vi "Format Numeric to String.vi"(6 "Numeric":dbl, 7 "Endian":T1, 8 "Format String":string, 9 "List":string[](array[string]), 10 "Channel Type":T2, 11 "Type":T3) -> (3 "Value":string)   [LabVIEW 2018, in "Instrument Addon Engine.lvlib"]
uses:
  Instrument Addon Engine.lvlib
  Addon Shared/Types/Type Cast Type.ctl
  Addon Shared/Types/Metadata Channel Type.ctl
  Addon Shared/Types/Endian.ctl
  Addon Shared/Instrument Addon Shared.lvlib
panel:
  in  "error in":errorcluster
  out "error out":errorcluster
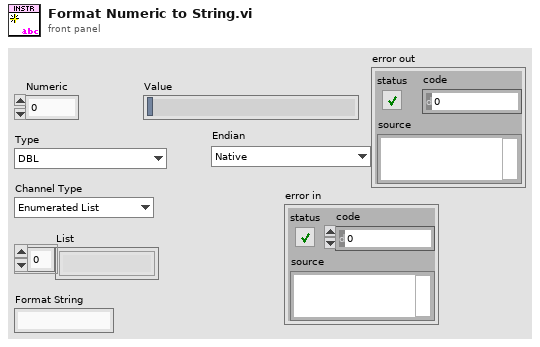
[diagram p1: front panel]
types:
  T1 = typedef "Instrument Addon Shared.lvlib/Endian.ctl" = enum16{"Native", "Little", "Big"}
  T2 = typedef "Instrument Addon Shared.lvlib/Metadata Channel Type.ctl" = enum16{"Enumerated List", "Format", "Type Cast"}
  T3 = typedef "Instrument Addon Shared.lvlib/Type Cast Type.ctl" = enum16{"DBL", "SGL", "U64", "U32", "U16", "U8", "I64", "I32", "I16", "I8"}
  T4 = enum16{"big-endian, network order", "native, host order", "little-endian"}
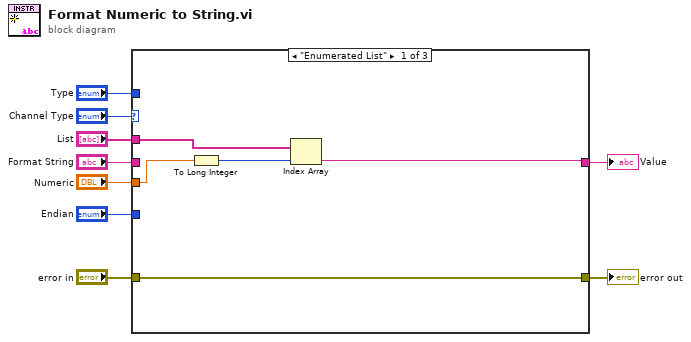
[diagram p0: block diagram]
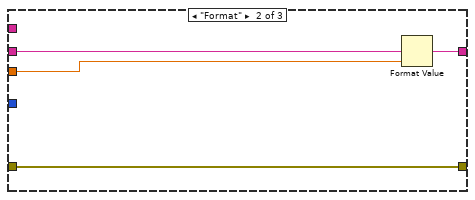
[diagram p2: hidden frame]
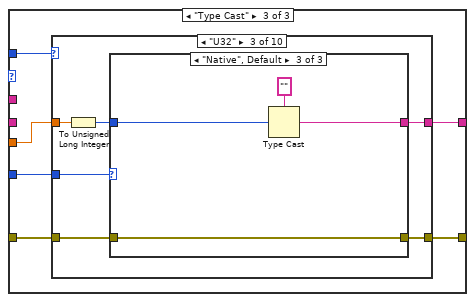
[diagram p3: hidden frame]
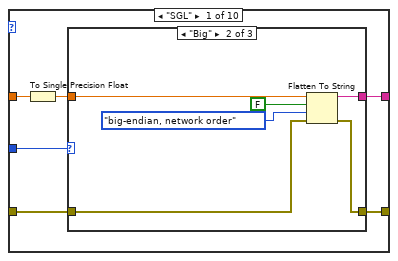
[diagram p4: hidden frame]
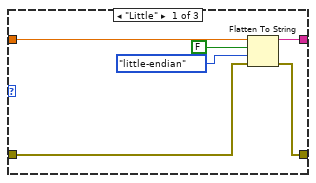
[diagram p5: hidden frame]
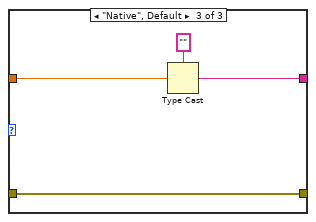
[diagram p6: hidden frame]
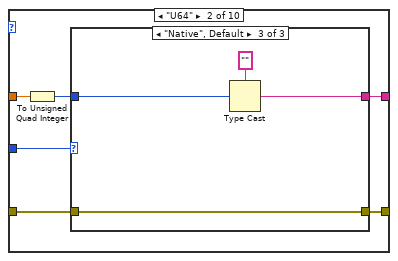
[diagram p7: hidden frame]
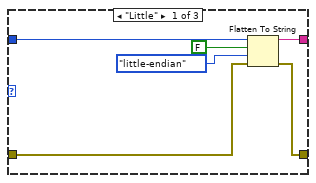
[diagram p8: hidden frame]
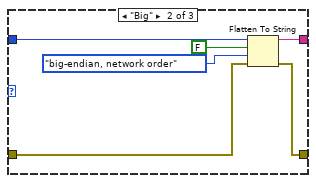
[diagram p9: hidden frame]
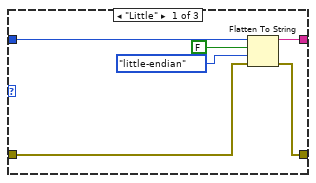
[diagram p10: hidden frame]
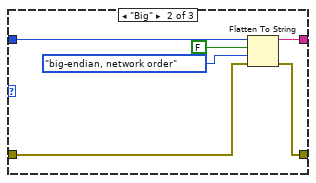
[diagram p11: hidden frame]
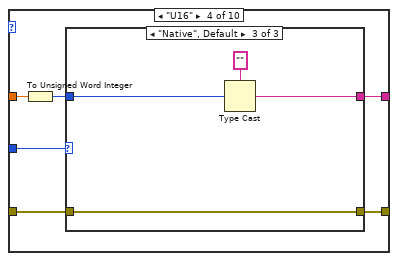
[diagram p12: hidden frame]
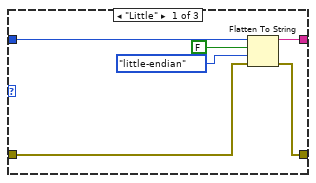
[diagram p13: hidden frame]
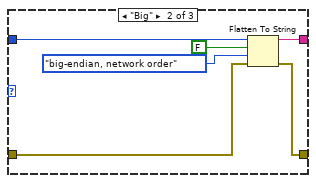
[diagram p14: hidden frame]
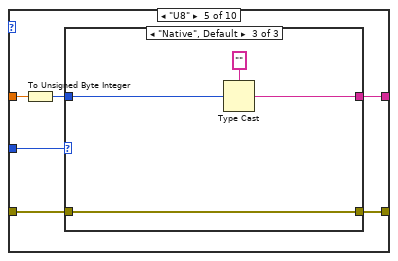
[diagram p15: hidden frame]
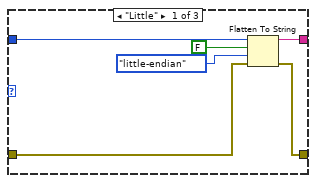
[diagram p16: hidden frame]
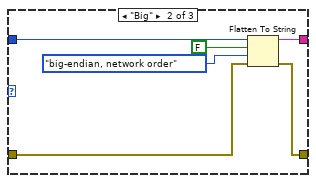
[diagram p17: hidden frame]
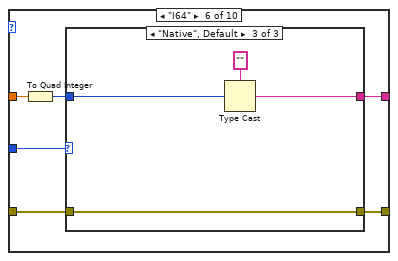
[diagram p18: hidden frame]
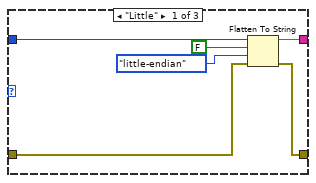
[diagram p19: hidden frame]
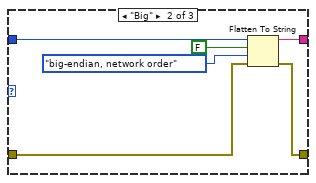
[diagram p20: hidden frame]
diagram:
  n1 = case shown="\"Enumerated List\"" "Channel Type" {
    tunnel: "List" -> [w14 _ _]
    tunnel: "Format String" -> [_ w18 _]
    tunnel: "Numeric" -> [w13 w17 w24]
    tunnel: [w11 w16 w23] -> w7
    tunnel: "Type" -> [_ _ w22]
    tunnel: "Endian" -> [_ _ w21]
    tunnel: [w10 w15 w20] -> w2
    tunnel: "error in" -> [w10 w15 w19]
    frame "Enumerated List" {
      n2 = To Long Integer(number=w13) -> (32bit integer=w12:i32)
      n3 = Index Array(array=w14, index=w12) -> (element=w11:string)
    }
    frame "Format" {
      n4 = Format Value(format string=w18, value (0)=w17) -> (output string=w16:string)  [unwired: 1 in]
    }
    frame "Type Cast" {
      n5 = case shown="\"U32\"" w22 {
        tunnel: w24 -> [w30 w52 w74 w96 w118 w140 w162 w184 w206 w225]
        tunnel: [w25 w48 w70 w91 w113 w135 w157 w183 w204 w224] -> w23
        tunnel: w21 -> [w28 w50 w73 w94 w116 w138 w160 w181 w201 w226]
        tunnel: [w26 w47 w69 w92 w114 w136 w158 w180 w203 w223] -> w20
        tunnel: w19 -> [w27 w51 w72 w93 w115 w137 w159 w179 w202 w227]
        frame "SGL" {
          n6 = To Single Precision Float(number=w30) -> (single precision float=w29:sgl)
          n7 = case shown="\"Big\"" w28 {
            tunnel: [w35 w41 w46] -> w25
            tunnel: w29 -> [w36 w42 w45]
            tunnel: [w33 w39 w43] -> w26
            tunnel: w27 -> [w32 w38 w43]
            frame "Little" {
              n8 = Flatten To String(anything=w36, prepend array or string size? (T)=FALSE, byte order (0:big-endian, network order)=T4."little-endian", error in (no error)=w32) -> (data string=w35:string, error out=w33:errorcluster)  [unwired: 1 out]
            }
            frame "Big" {
              n9 = Flatten To String(anything=w42, prepend array or string size? (T)=FALSE, byte order (0:big-endian, network order)=T4."big-endian, network order", error in (no error)=w38) -> (data string=w41:string, error out=w39:errorcluster)  [unwired: 1 out]
            }
            frame "Native", Default {
              n10 = Type Cast(type="", x=w45) -> (*(type *) &x=w46:string)
            }
          }
        }
        frame "U64" {
          n11 = To Unsigned Quad Integer(1:w52) -> (0:w49:u64)
          n12 = case shown="\"Native\", Default" w50 {
            tunnel: [w57 w63 w68] -> w48
            tunnel: w49 -> [w58 w64 w67]
            tunnel: [w55 w61 w65] -> w47
            tunnel: w51 -> [w54 w60 w65]
            frame "Little" {
              n13 = Flatten To String(anything=w58, prepend array or string size? (T)=FALSE, byte order (0:big-endian, network order)=T4."little-endian", error in (no error)=w54) -> (data string=w57:string, error out=w55:errorcluster)  [unwired: 1 out]
            }
            frame "Big" {
              n14 = Flatten To String(anything=w64, prepend array or string size? (T)=FALSE, byte order (0:big-endian, network order)=T4."big-endian, network order", error in (no error)=w60) -> (data string=w63:string, error out=w61:errorcluster)  [unwired: 1 out]
            }
            frame "Native", Default {
              n15 = Type Cast(type="", x=w67) -> (*(type *) &x=w68:string)
            }
          }
        }
        frame "U32" {
          n16 = To Unsigned Long Integer(number=w74) -> (unsigned 32bit integer=w71:u32)
          n17 = case shown="\"Native\", Default" w73 {
            tunnel: [w79 w85 w90] -> w70
            tunnel: w71 -> [w80 w86 w89]
            tunnel: [w77 w83 w87] -> w69
            tunnel: w72 -> [w76 w82 w87]
            frame "Little" {
              n18 = Flatten To String(anything=w80, prepend array or string size? (T)=FALSE, byte order (0:big-endian, network order)=T4."little-endian", error in (no error)=w76) -> (data string=w79:string, error out=w77:errorcluster)  [unwired: 1 out]
            }
            frame "Big" {
              n19 = Flatten To String(anything=w86, prepend array or string size? (T)=FALSE, byte order (0:big-endian, network order)=T4."big-endian, network order", error in (no error)=w82) -> (data string=w85:string, error out=w83:errorcluster)  [unwired: 1 out]
            }
            frame "Native", Default {
              n20 = Type Cast(type="", x=w89) -> (*(type *) &x=w90:string)
            }
          }
        }
        frame "U16" {
          n21 = To Unsigned Word Integer(number=w96) -> (unsigned 16bit integer=w95:u16)
          n22 = case shown="\"Native\", Default" w94 {
            tunnel: [w101 w107 w112] -> w91
            tunnel: w95 -> [w102 w108 w111]
            tunnel: [w99 w105 w109] -> w92
            tunnel: w93 -> [w98 w104 w109]
            frame "Little" {
              n23 = Flatten To String(anything=w102, prepend array or string size? (T)=FALSE, byte order (0:big-endian, network order)=T4."little-endian", error in (no error)=w98) -> (data string=w101:string, error out=w99:errorcluster)  [unwired: 1 out]
            }
            frame "Big" {
              n24 = Flatten To String(anything=w108, prepend array or string size? (T)=FALSE, byte order (0:big-endian, network order)=T4."big-endian, network order", error in (no error)=w104) -> (data string=w107:string, error out=w105:errorcluster)  [unwired: 1 out]
            }
            frame "Native", Default {
              n25 = Type Cast(type="", x=w111) -> (*(type *) &x=w112:string)
            }
          }
        }
        frame "U8" {
          n26 = To Unsigned Byte Integer(number=w118) -> (unsigned 8bit integer=w117:u8)
          n27 = case shown="\"Native\", Default" w116 {
            tunnel: [w123 w129 w134] -> w113
            tunnel: w117 -> [w124 w130 w133]
            tunnel: [w121 w127 w131] -> w114
            tunnel: w115 -> [w120 w126 w131]
            frame "Little" {
              n28 = Flatten To String(anything=w124, prepend array or string size? (T)=FALSE, byte order (0:big-endian, network order)=T4."little-endian", error in (no error)=w120) -> (data string=w123:string, error out=w121:errorcluster)  [unwired: 1 out]
            }
            frame "Big" {
              n29 = Flatten To String(anything=w130, prepend array or string size? (T)=FALSE, byte order (0:big-endian, network order)=T4."big-endian, network order", error in (no error)=w126) -> (data string=w129:string, error out=w127:errorcluster)  [unwired: 1 out]
            }
            frame "Native", Default {
              n30 = Type Cast(type="", x=w133) -> (*(type *) &x=w134:string)
            }
          }
        }
        frame "I64" {
          n31 = To Quad Integer(1:w140) -> (0:w139:i64)
          n32 = case shown="\"Native\", Default" w138 {
            tunnel: [w145 w151 w156] -> w135
            tunnel: w139 -> [w146 w152 w155]
            tunnel: [w143 w149 w153] -> w136
            tunnel: w137 -> [w142 w148 w153]
            frame "Little" {
              n33 = Flatten To String(anything=w146, prepend array or string size? (T)=FALSE, byte order (0:big-endian, network order)=T4."little-endian", error in (no error)=w142) -> (data string=w145:string, error out=w143:errorcluster)  [unwired: 1 out]
            }
            frame "Big" {
              n34 = Flatten To String(anything=w152, prepend array or string size? (T)=FALSE, byte order (0:big-endian, network order)=T4."big-endian, network order", error in (no error)=w148) -> (data string=w151:string, error out=w149:errorcluster)  [unwired: 1 out]
            }
            frame "Native", Default {
              n35 = Type Cast(type="", x=w155) -> (*(type *) &x=w156:string)
            }
          }
        }
        frame "I32" {
          n36 = To Long Integer(number=w162) -> (32bit integer=w161:i32)
          n37 = case shown="\"Little\"" w160 {
            tunnel: [w167 w173 w178] -> w157
            tunnel: w161 -> [w168 w174 w177]
            tunnel: [w165 w171 w175] -> w158
            tunnel: w159 -> [w164 w170 w175]
            frame "Little" {
              n38 = Flatten To String(anything=w168, prepend array or string size? (T)=FALSE, byte order (0:big-endian, network order)=T4."little-endian", error in (no error)=w164) -> (data string=w167:string, error out=w165:errorcluster)  [unwired: 1 out]
            }
            frame "Big" {
              n39 = Flatten To String(anything=w174, prepend array or string size? (T)=FALSE, byte order (0:big-endian, network order)=T4."big-endian, network order", error in (no error)=w170) -> (data string=w173:string, error out=w171:errorcluster)  [unwired: 1 out]
            }
            frame "Native", Default {
              n40 = Type Cast(type="", x=w177) -> (*(type *) &x=w178:string)
            }
          }
        }
        frame "I16" {
          n41 = To Word Integer(number=w184) -> (16bit integer=w182:i16)
          n42 = case shown="\"Native\", Default" w181 {
            tunnel: [w189 w195 w200] -> w183
            tunnel: w182 -> [w190 w196 w199]
            tunnel: [w187 w193 w197] -> w180
            tunnel: w179 -> [w186 w192 w197]
            frame "Little" {
              n43 = Flatten To String(anything=w190, prepend array or string size? (T)=FALSE, byte order (0:big-endian, network order)=T4."little-endian", error in (no error)=w186) -> (data string=w189:string, error out=w187:errorcluster)  [unwired: 1 out]
            }
            frame "Big" {
              n44 = Flatten To String(anything=w196, prepend array or string size? (T)=FALSE, byte order (0:big-endian, network order)=T4."big-endian, network order", error in (no error)=w192) -> (data string=w195:string, error out=w193:errorcluster)  [unwired: 1 out]
            }
            frame "Native", Default {
              n45 = Type Cast(type="", x=w199) -> (*(type *) &x=w200:string)
            }
          }
        }
        frame "I8" {
          n46 = To Byte Integer(number=w206) -> (8bit integer=w205:i8)
          n47 = case shown="\"Big\"" w201 {
            tunnel: [w211 w217 w222] -> w204
            tunnel: w205 -> [w212 w218 w221]
            tunnel: [w209 w215 w219] -> w203
            tunnel: w202 -> [w208 w214 w219]
            frame "Little" {
              n48 = Flatten To String(anything=w212, prepend array or string size? (T)=FALSE, byte order (0:big-endian, network order)=T4."little-endian", error in (no error)=w208) -> (data string=w211:string, error out=w209:errorcluster)  [unwired: 1 out]
            }
            frame "Big" {
              n49 = Flatten To String(anything=w218, prepend array or string size? (T)=FALSE, byte order (0:big-endian, network order)=T4."big-endian, network order", error in (no error)=w214) -> (data string=w217:string, error out=w215:errorcluster)  [unwired: 1 out]
            }
            frame "Native", Default {
              n50 = Type Cast(type="", x=w221) -> (*(type *) &x=w222:string)
            }
          }
        }
        frame "DBL" {
          n51 = case shown="\"Native\", Default" w226 {
            tunnel: [w232 w238 w243] -> w224
            tunnel: w225 -> [w233 w239 w242]
            tunnel: [w230 w236 w240] -> w223
            tunnel: w227 -> [w229 w235 w240]
            frame "Little" {
              n52 = Flatten To String(anything=w233, prepend array or string size? (T)=FALSE, byte order (0:big-endian, network order)=T4."little-endian", error in (no error)=w229) -> (data string=w232:string, error out=w230:errorcluster)  [unwired: 1 out]
            }
            frame "Big" {
              n53 = Flatten To String(anything=w239, prepend array or string size? (T)=FALSE, byte order (0:big-endian, network order)=T4."big-endian, network order", error in (no error)=w235) -> (data string=w238:string, error out=w236:errorcluster)  [unwired: 1 out]
            }
            frame "Native", Default {
              n54 = Type Cast(type="", x=w242) -> (*(type *) &x=w243:string)
            }
          }
        }
      }
    }
  }
  "Value" <- w7
  "error out" <- w2
